vi "Core Action.vi"(8 "error in (no error)":errorcluster, 10 "SECS-II Class":refnum<class "SECS-II Class.lvclass">, 11 "21-Material Movement in":refnum<class "21-Material Movement.lvclass">) -> (0 "error out":errorcluster, 2 "SECS-II Class Out":refnum<class "SECS-II Class.lvclass">, 3 "21-Material Movement out":refnum<class "21-Material Movement.lvclass">)   [LabVIEW 2020, in "SECS Scenarios.lvlib" / "21-Material Movement.lvclass"]
uses:
  21-Material Movement.lvclass
  D:/Dropbox/SECS/SECS_GEM v1.1.0/Com/SECS Scenarios/Scenarios Class/Scenarios Class.lvclass
  SECS Communication/SECS-II Class/SECS-II Class.lvclass
  21-Material Movement.lvclass/21-Material Movement.ctl
  Scenarios Class/Scenarios Class.lvclass
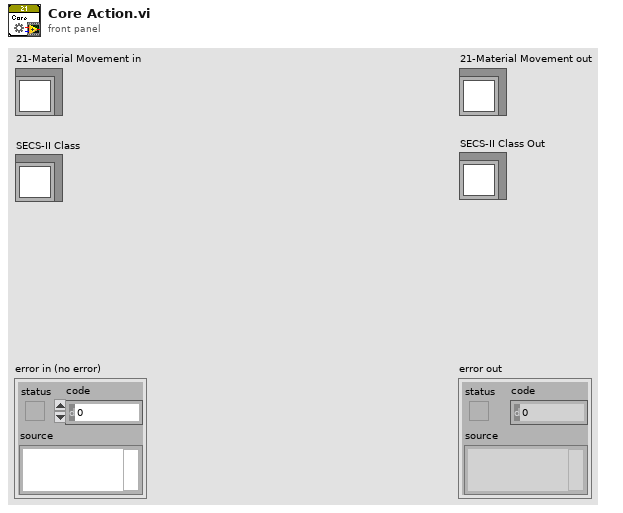
[diagram p1: front panel]
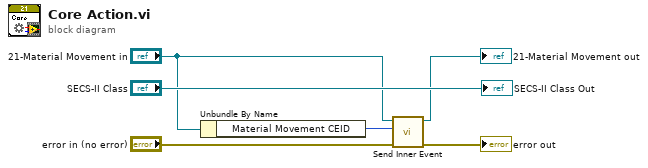
[diagram p0: block diagram]
diagram:
  n1 = Unbundle By Name("21-Material Movement in") -> ("Material Movement CEID"=w2:u32)
  n2 = call "Send Inner Event.vi"("error in (no error)"="error in (no error)", "CEID"=w2, "Scenarios Class in"="21-Material Movement in") -> ("error out"=→"error out":errorcluster, "Scenarios Class out"=→"21-Material Movement out":refnum<class "21-Material Movement.lvclass">)  [unwired: 7 in]
  "SECS-II Class Out" <- "SECS-II Class"
